vi "Module Timeout--constant.vi"() -> (3 "Module Timeout":i32)   [LabVIEW 2023, in "horiba.lvlib" / "DeviceManager.lvlib"]
doc: "A module-wide common value to use as the timeout for various synchronization actions.\n_____\nBased on DQMH Project Template 7.0.0.1280."
uses:
  DeviceManager.lvlib
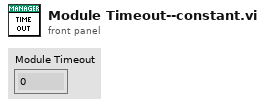
[diagram p1: front panel]
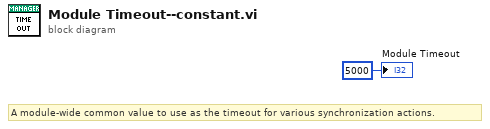
[diagram p0: block diagram]
diagram:
  # "A module-wide common value to use as the timeout for various synchronization actions."
  "Module Timeout" <- 5000 ("Module Timeout")
